vi "to test.vi"(8 "error in (no error)":errorcluster, 11 "Si UI in":refnum<class "Si UI.lvclass">) -> (0 "error out":errorcluster, 3 "Si UI out":refnum<class "Si UI.lvclass">)   [LabVIEW 2020, in "Si UI.lvlib" / "Si UI.lvclass"]
uses:
  Si UI.lvclass
  Si UI.lvclass/Si UI.ctl
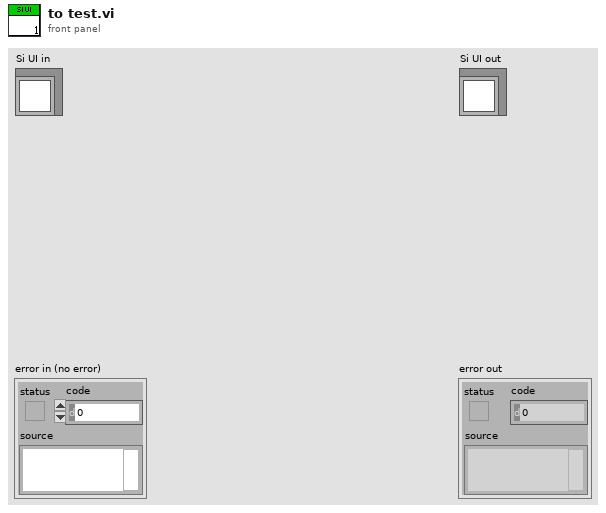
[diagram p1: front panel]
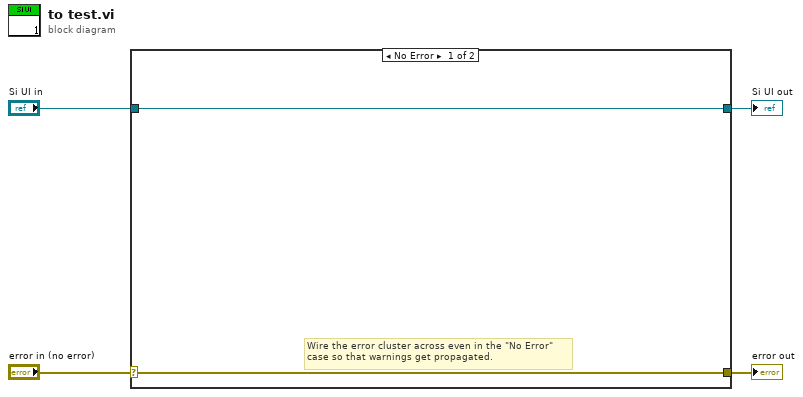
[diagram p0: block diagram]
diagram:
  n1 = case shown="No Error" "error in (no error)" {
    selector: "error in (no error)" -> [w5 w8]
    tunnel: [w5 w8] -> w3
    tunnel: [w6 w7] -> w1
    tunnel: "Si UI in" -> [w6 w7]
    frame No Error {
      # "Wire the error cluster across even in the \"No Error\"\ncase so that warnings get propagated."
    }
    frame Error {
    }
  }
  "error out" <- w3
  "Si UI out" <- w1
